vi "Snap.vi"(8 "error in (no error)":errorcluster, 11 "Camera in":refnum<class "Camera.lvclass">) -> (0 "error out":errorcluster, 2 "SnapInfo":T1, 3 "Camera out":refnum<class "Camera.lvclass">)   [LabVIEW 2020, in "CameraUSB.lvlib" / "Camera.lvclass"]
uses:
  Camera.lvclass
  ICamera/TypeDef/SnapInfo.ctl
  Camera.lvclass/Camera.ctl
  ICamera/TypeDef/ICamera_typedef.lvlib
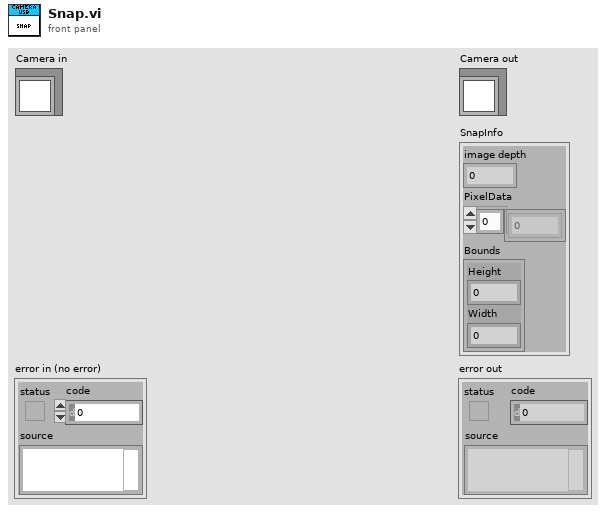
[diagram p1: front panel]
types:
  T1 = typedef "ICamera_typedef.lvlib/SnapInfo.ctl" = cluster{"image depth":i32, "PixelData":u8[], "Bounds":cluster{"Height":i16, "Width":i16}}
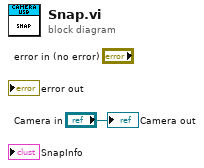
[diagram p0: block diagram]
diagram:
  "Camera out" <- "Camera in"
